vi "Door Status Global Variable.vi"() -> ()   [LabVIEW 2018]
panel:
  in  "Cable In Use":bool
  in  "stop":bool
  in  "Door Status":bool
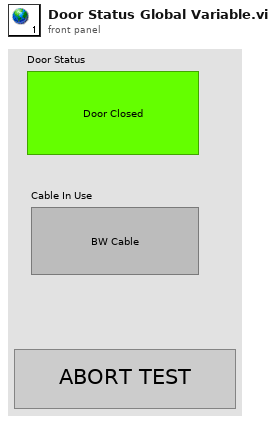
[diagram p1: front panel]
diagram:
